vi "Write Run_.vi"(8 "error in (no error)":errorcluster, 10 "Run?":bool, 11 "Change O3 Lamp Run MSG in":refnum<class "Change O3 Lamp Run MSG.lvclass">) -> (0 "error out":errorcluster, 3 "Change O3 Lamp Run MSG out":refnum<class "Change O3 Lamp Run MSG.lvclass">)   [LabVIEW 2014, in "Change O3 Lamp Run MSG.lvclass"]
uses:
  Change O3 Lamp Run MSG.lvclass
  Change O3 Lamp Run MSG.lvclass/Change O3 Lamp Run MSG.ctl
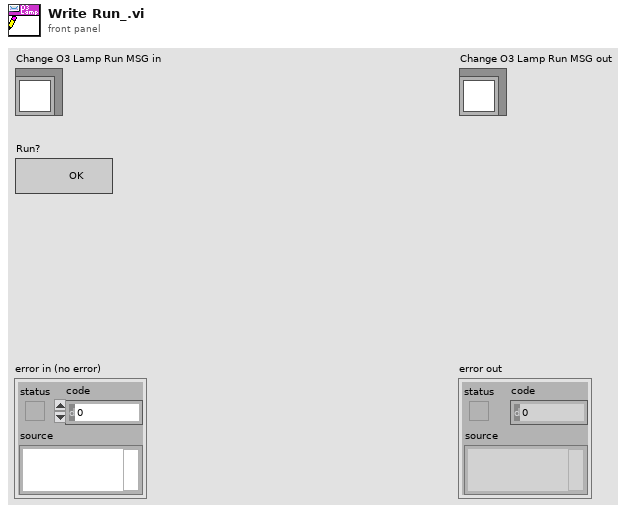
[diagram p1: front panel]
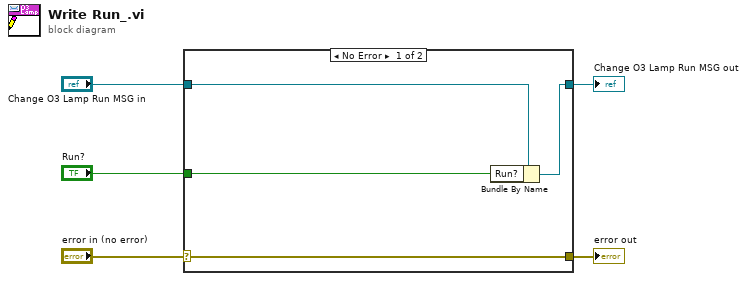
[diagram p0: block diagram]
diagram:
  n1 = case shown="No Error" "error in (no error)" {
    selector: "error in (no error)" -> [w9 w10]
    tunnel: [w9 w10] -> w4
    tunnel: [w7 w11] -> w2
    tunnel: "Change O3 Lamp Run MSG in" -> [w8 w11]
    tunnel: "Run?" -> [w6 _]
    frame No Error {
      n2 = Bundle By Name(cluster=w8, "Run?"=w6) -> (w7:refnum<class "Change O3 Lamp Run MSG.lvclass">)
    }
    frame Error {
    }
  }
  "error out" <- w4
  "Change O3 Lamp Run MSG out" <- w2
